vi "CSATKdll.vi"(8 "error in (no error)":errorcluster, 11 "Inputs":cluster{"icomp":i32, "t":dbl, "kph":i32}) -> (0 "error out":errorcluster, 3 "Outputs":T1)   [LabVIEW 2016]
doc: "subroutine CSATKdll(icomp, t, kph, p, d, csat, ierr, herr, herr_length)\n\nCompute the heat capacity along the saturation line as a function of temperature for a given component.\nCsat can be calculated in several ways: Csat = T*(dS/dT[sat]) Csat = Cp - T*(dV/dT)(dP/dT[sat]) with dVdT at\nconstant pressure Csat = Cp - beta/D*hvap/(vliq - vvap) where beta is the volume expansivity\n\nINPUTS:\nicomp -- Component number in mixture (1..nc); 1 for pure fluid\nt -- Temperature [K]\nkph -- Phase flag: 1 - Liquid calculation 2 - Vapor calculation\n\nOUTPUTS:\np -- Saturated pressure [kPa]\nd -- Saturated molar density [mol/L]\ncsat -- Saturated heat capacity [J/mol-K]\nierr -- Error flag: 0 = Successful\nherr -- Error string (character*255)\nherr_length -- length of variable herr (default: 255)"
uses:
  REFPROP.DLL
panel:
  # "REFPROP-CSATKdll.vi"
  # "void  CSATKdll(int32_t *icomp, double *t, int32_t *kph, double *p, double *d, double *csat, int32_t *ierr, CStr herr, int32_t herr_length)"
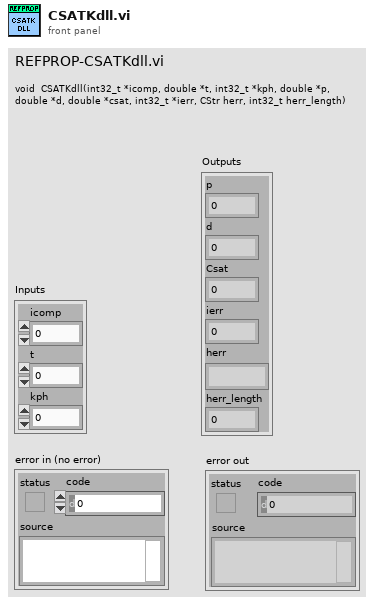
[diagram p1: front panel]
types:
  T1 = cluster{"p":dbl, "d":dbl, "Csat":dbl, "ierr":i32, "herr":string, "herr_length":i32}
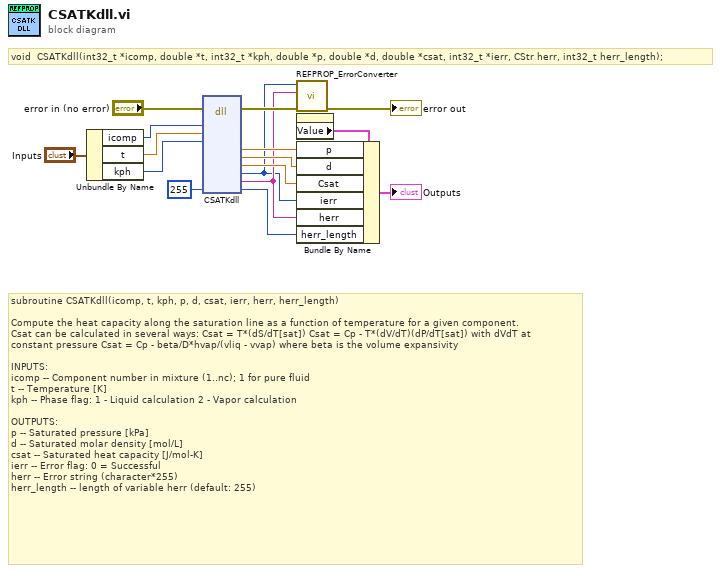
[diagram p0: block diagram]
diagram:
  # "void  CSATKdll(int32_t *icomp, double *t, int32_t *kph, double *p, double *d, double *csat, int32_t *ierr, CStr herr, int32_t herr_length);"
  # "subroutine CSATKdll(icomp, t, kph, p, d, csat, ierr, herr, herr_length)\n\nCompute the heat capacity along the saturation line as a function of temperature for a given component.\nCsat can be calculated in several ways: Csat = T*(dS/dT[sat]) Csat = Cp - T*(dV/dT)(dP/dT[sat]) with dVdT at\nconstant pressure Csat = Cp - beta/D*hvap/(vliq - vvap) where beta is the volume expansivity\n\nINPUTS:\nicomp -- Component number in mixture (1..nc); 1 for pure fluid\nt -- Temperature [K]\nkph -- Phase flag: 1 - Liquid calculation 2 - Vapor calculation\n\nOUTPUTS:\np -- Saturated pressure [kPa]\nd -- Saturated molar density [mol/L]\ncsat -- Saturated heat capacity [J/mol-K]\nierr -- Error flag: 0 = Successful\nherr -- Error string (character*255)\nherr_length -- length of variable herr (default: 255)"
  n1 = Unbundle By Name("Inputs") -> ("icomp"=w11:i32, "t"=w10:dbl, "kph"=w9:i32)
  n2 = dll-call lib="S:/009 - Testing/02 - Performance Testing/REFPROP/REFPROP.*" fn="CSATKdll"(error in="error in (no error)", "icomp"=w11, "t"=w10, "kph"=w9, "herr_length"=255) -> (error out=w15:errorcluster, "p"=w6:dbl, "d"=w3:dbl, "csat"=w4:dbl, "ierr"=w1:i32, "herr"=w2:string, "herr_length"=w5:i32)  [unwired: 11 in, 1 out]
  n3 = call "REFPROP_ErrorConverter.vi"("error in (no error)"=w15, "Error Message"=w2, "Error Code"=w1) -> ("error out"=→"error out":errorcluster)  [unwired: 8 in]
  n4 = property on="Outputs" class="Clust (strict)"() -> ("Value"=w8:T1)  [unwired: 2 in, 2 out]
  n5 = Bundle By Name(cluster=w8, "p"=w6, "d"=w3, "Csat"=w4, "ierr"=w1, "herr"=w2, "herr_length"=w5) -> (→"Outputs":T1)
